vi "Check if LogFile Exists.vi"(7 "System Definition Path":path, 8 "error in (no error)":errorcluster, 11 "Target Refnum in":refnum<k24>) -> (0 "error out":errorcluster, 3 "Target Refnum out":refnum<k24>, 5 "LogFile Exists?":bool)   [LabVIEW 2019, in "TLCD System Tests.lvclass"]
uses:
  TLCD System Tests.lvclass
  NationalInstruments.VeriStand.SystemDefinitionAPI
  TLCD Test Class/TLCD Test Class.lvclass
  <vilib>/WebDAVClient/NI_WebDAV.lvlib
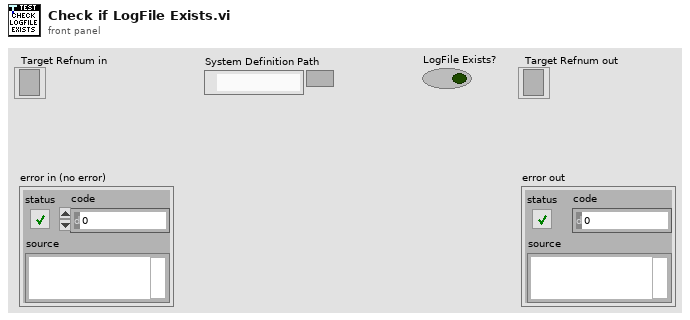
[diagram p1: front panel]
types:
  T1 = typedef "NI_WebDAV.lvlib/SessionHandle.ctl" = refnum<k1>
  T2 = typedef "NI_WebDAV.lvlib/FileInfo.ctl" = cluster{"type":string, "size":u64, "last modification":timestamp, "display name":string, "uri":string}
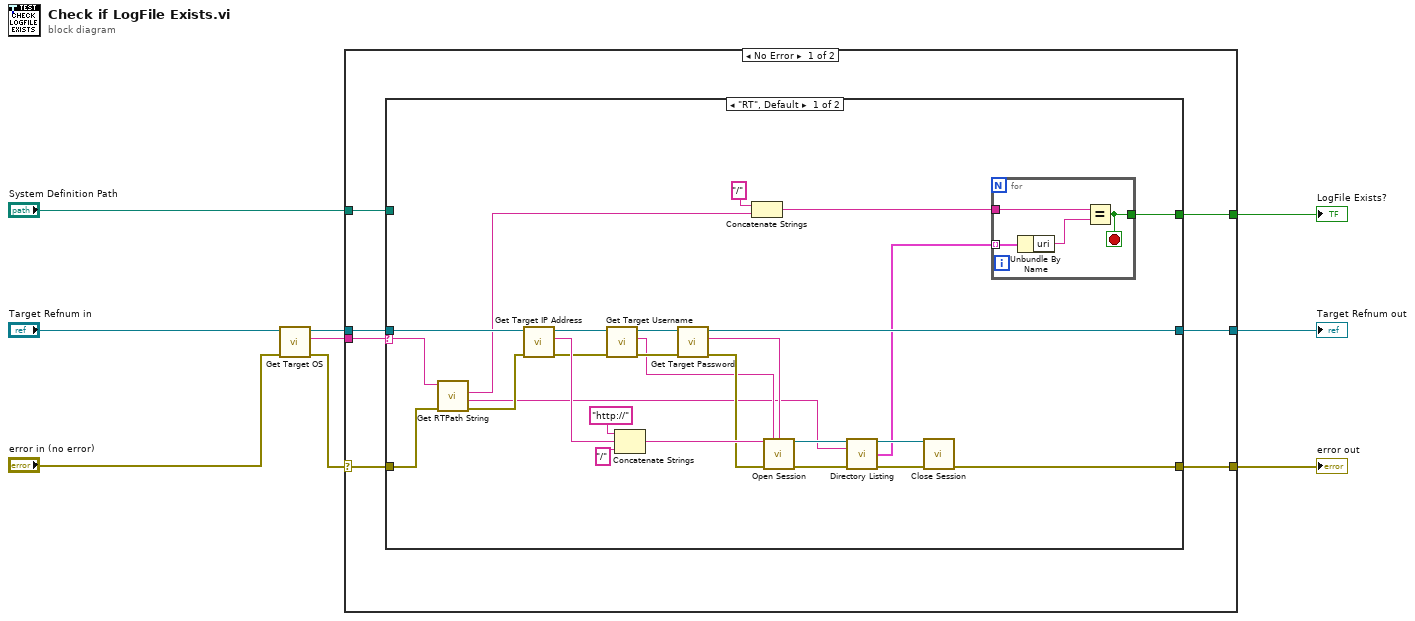
[diagram p0: block diagram]
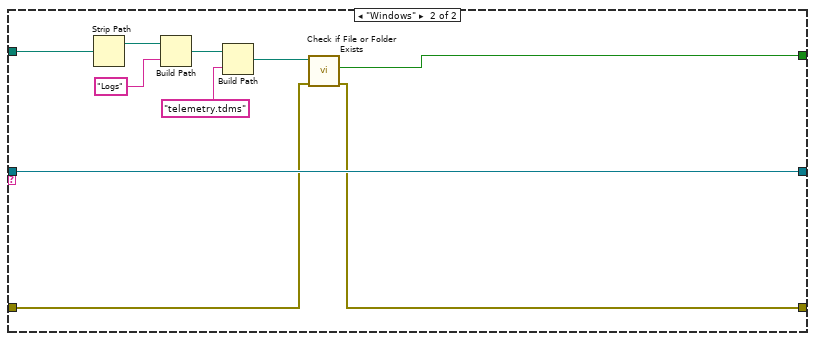
[diagram p2: hidden frame]
diagram:
  n1 = call "Get Target OS.vi"("error in (no error)"="error in (no error)", "Target ref in"="Target Refnum in") -> ("error out"=w1:errorcluster, "OperatingSystem"=w7:string, "Target ref out"=w6:refnum<k24>)  [unwired: 7 in]
  n2 = case shown="No Error" w1 {
    selector: w1 -> [w10 w59]
    tunnel: [w16 _] -> w9
    tunnel: "System Definition Path" -> [w15 _]
    tunnel: w7 -> [w14 _]
    tunnel: w6 -> [w13 w58]
    tunnel: [w12 w58] -> w3
    tunnel: [w11 w59] -> w2
    frame No Error {
      n3 = case shown="\"RT\", Default" w14 {
        selector: w14 -> [w43 _]
        tunnel: [w25 w49] -> w11
        tunnel: [w26 w57] -> w12
        tunnel: w10 -> [w42 w50]
        tunnel: w13 -> [w41 w57]
        tunnel: w15 -> [_ w56]
        tunnel: [w17 w48] -> w16
        frame "RT", Default {
          n4 = call "Get RTPath String.vi"("error in (no error)"=w42, "Target OS in"=w43) -> ("error out"=w40:errorcluster, "RT Folder Path"=w22:string, "RT File Path"=w20:string)  [unwired: 6 in, 1 out]
          n5 = call "Get Target IP Address.vi"("error in (no error)"=w40, "Target ref in"=w41) -> ("error out"=w33:errorcluster, "IPAddress"=w38:string, "Target ref out"=w35:refnum<k24>)  [unwired: 7 in]
          n6 = call "Get Target Username.vi"("error in (no error)"=w33, "Target ref in"=w35) -> ("error out"=w32:errorcluster, "Username"=w29:string, "Target ref out"=w34:refnum<k24>)  [unwired: 7 in]
          n7 = Concatenate Strings("http://" ("string"), w38, "/" ("string")) -> (w36:string)
          n8 = call "Get Target Password.vi"("error in (no error)"=w32, "Target ref in"=w34) -> ("error out"=w31:errorcluster, "Password"=w30:string, "Target ref out"=w26:refnum<k24>)  [unwired: 7 in]
          n9 = Concatenate Strings("/" ("string"), w20) -> (w19:string)
          n10 = call <vilib>:"Open Session.vi"("host uri prefix"=w36, "username"=w29, "password"=w30, "error in (no error)"=w31) -> ("session handle out"=w27:T1, "error out"=w28:errorcluster)  [unwired: 10 in]
          n11 = call <vilib>:"Directory Listing.vi"("session handle"=w27, "relative uri"=w22, "error in (no error)"=w28) -> ("session handle out"=w24:T1, "file list"=w21:T2[], "error out"=w23:errorcluster)  [unwired: 9 in, 1 out]
          n12 = call <vilib>:"Close Session.vi"("session handle"=w24, "error in (no error)"=w23) -> ("error out"=w25:errorcluster)  [unwired: 13 in]
          n13 = for {
            tunnel: w21 -> [w47] mode=indexing
            tunnel: w19 -> [w45]
            tunnel: [w44] -> w17
            stop <- w44 stop-if-true
            n14 = Unbundle By Name(w47) -> ("uri"=w46:string)
            n15 = Equal?(x=w45, y=w46) -> (x = y?=w44:bool)
          }
        }
        frame "Windows" {
          n16 = Strip Path(path=w56) -> (stripped path=w55:path)  [unwired: 1 out]
          n17 = Build Path(base path=w55, name or relative path="Logs") -> (appended path=w53:path)
          n18 = Build Path(base path=w53, name or relative path="telemetry.tdms") -> (appended path=w51:path)
          n19 = call <vilib>:"Check if File or Folder Exists.vi"("error in (no error)"=w50, "path"=w51) -> ("error out"=w49:errorcluster, "file or folder exists?"=w48:bool)  [unwired: 7 in, 1 out]
        }
      }
    }
    frame Error {
    }
  }
  "LogFile Exists?" <- w9
  "Target Refnum out" <- w3
  "error out" <- w2
